vi "tlc_Hardware Module.vi"(7 "Command (Write)":T1=enum."Write", 8 "error in (no error)":errorcluster, 9 "Color":u32(colorbox), 10 "Intensity":u32, 11 "Channel":u32) -> (0 "error out":errorcluster)   [LabVIEW 2010]
uses:
  tlc_Hardware_Command Control.ctl
panel:
  # "Input Data"
  # "Local Data"
  # "Output Data"
  # "No Local Data"
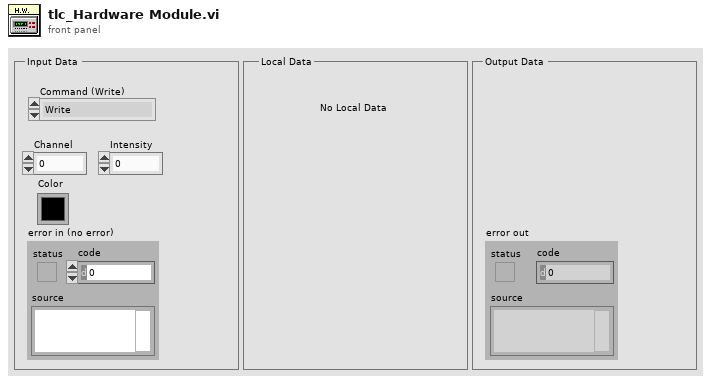
[diagram p1: front panel]
types:
  T1 = typedef "tlc_Hardware_Command Control.ctl" = enum16{"Initialize", "Write", "Shutdown"}
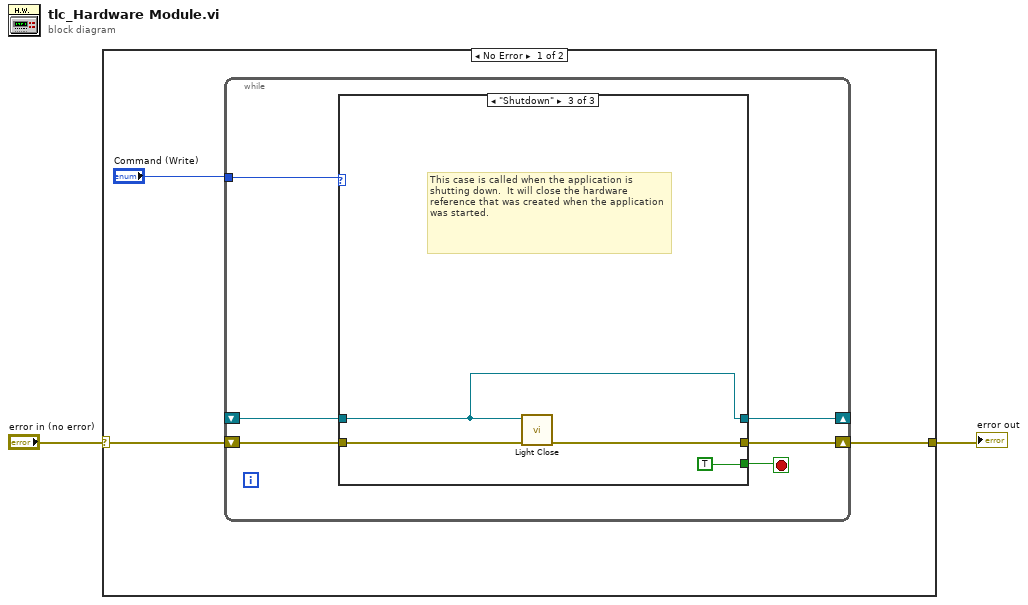
[diagram p0: block diagram]
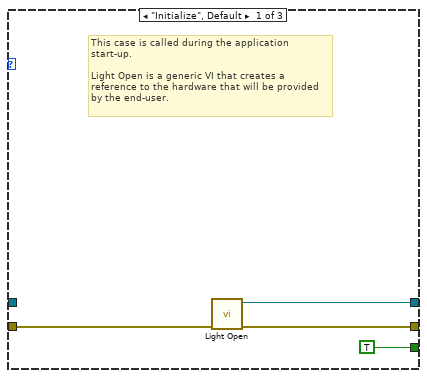
[diagram p2: hidden frame]
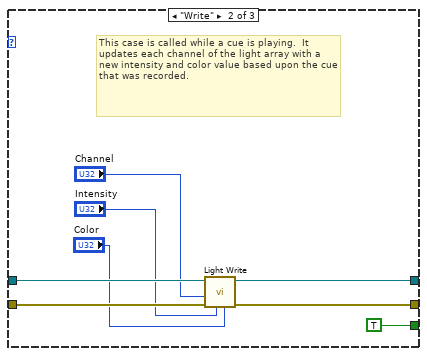
[diagram p3: hidden frame]
diagram:
  n1 = case shown="No Error" "error in (no error)" {
    selector: "error in (no error)" -> [w5 w28]
    tunnel: [w4 w28] -> w1
    frame No Error {
      n2 = while {
        shift-right: [w9] -> w4
        shift-left: w5 -> [w10]
        shift-right: [w8] -> _
        shift-left: _ -> [w7]
        tunnel: "Command (Write)" -> [w6]
        stop <- w11 stop-if-true
        n3 = case shown="\"Shutdown\"" w6 {
          tunnel: [TRUE TRUE TRUE] -> w11
          tunnel: w10 -> [w14 w23 w26]
          tunnel: [w13 w21 w25] -> w9
          tunnel: [w12 w16 w24] -> w8
          tunnel: w7 -> [_ w20 w24]
          frame "Initialize", Default {
            # "This case is called during the application start-up. \n\nLight Open is a generic VI that creates a reference to the hardware that will be provided by the end-user."
            n4 = call "Light Open.vi"("error in (no error)"=w14) -> ("error out"=w13:errorcluster, "Lighting Refnum"=w12:refnum<k1>)  [unwired: 8 in]
          }
          frame "Write" {
            # "This case is called while a cue is playing.  It updates each channel of the light array with a new intensity and color value based upon the cue that was recorded."
            n5 = call "Light Write.vi"("Color"="Color", "Intensity"="Intensity", "error in (no error)"=w23, "Channel"="Channel", "Lighting Refnum In"=w20) -> ("error out"=w21:errorcluster, "Lighting Refnum Out"=w16:refnum<k1>)  [unwired: 5 in]
          }
          frame "Shutdown" {
            # "This case is called when the application is shutting down.  It will close the hardware reference that was created when the application was started."
            n6 = call "Light Close.vi"("error in (no error)"=w26, "Lighting Refnum In"=w24) -> ("error out"=w25:errorcluster)  [unwired: 9 in]
          }
        }
      }
    }
    frame Error {
    }
  }
  "error out" <- w1
